vi "AutoWaitForArm_ORIG.vi"(8 "error in (no error)":errorcluster, 11 "TimeOut (s)":dbl=5.0) -> (0 "error out":errorcluster)   [LabVIEW 2020]
doc: "Wrapper class for auto do nothing and wait\nInput:\n -- error in -- Cluster \n -- time out -- Double -- how long to wait B4 quitting\nOutput:\n -- error out -- Cluster"
uses:
  <vilib>/Utility/semaphor.llb/Obtain Semaphore Reference.vi
  <vilib>/Rock Robotics/WPI/ThirdParty/JAS_Junk/TrajLib/Timer_Reset.vi
  <vilib>/Rock Robotics/WPI/ThirdParty/JAS_Junk/TrajLib/Trajectory_Library.lvlib
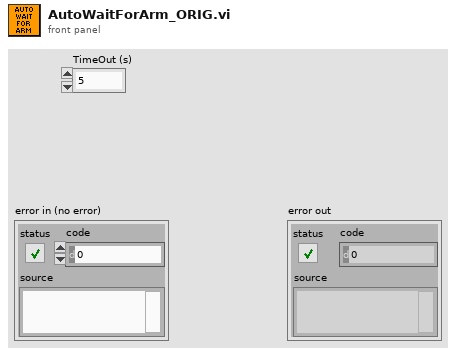
[diagram p1: front panel]
types:
  T1 = typedef "Trajectory_Library.lvlib/TIMER.ctl" = cluster{"StartTime":dbl, "Accumulated TIme":dbl, "Running":bool, "semaphore":T2}
  T2 = typedef "Semaphore RefNum" = refnum<k1>
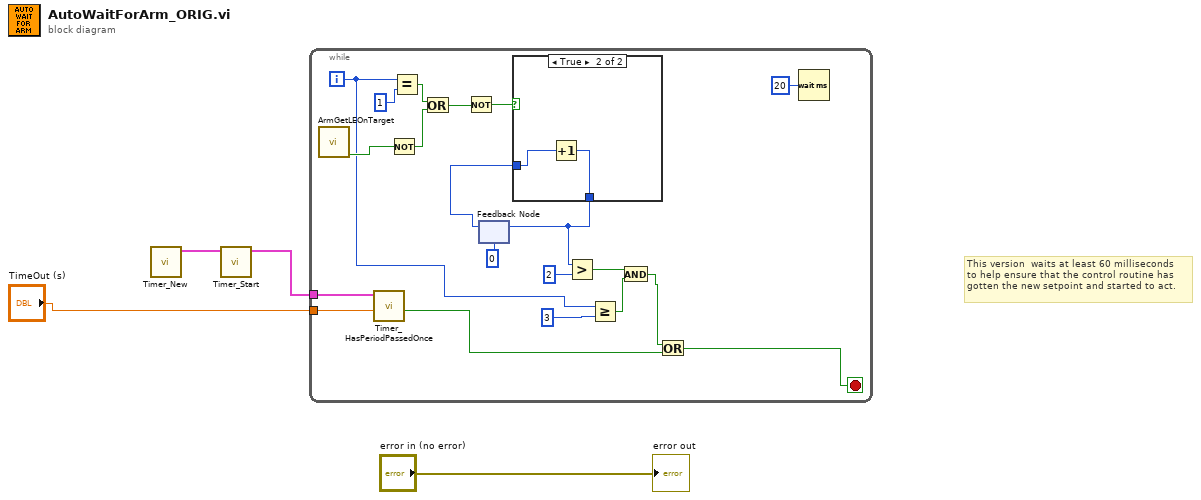
[diagram p0: block diagram]
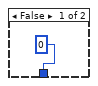
[diagram p2: hidden frame]
diagram:
  # "This version  waits at least 60 milliseconds\nto help ensure that the control routine has\ngotten the new setpoint and started to act."
  n1 = call <vilib>:"Timer_New.vi"() -> ("TIMER"=w3:T1)  [unwired: 11 in]
  n2 = call <vilib>:"Timer_Start.vi"("in Timer"=w3) -> ("out Timer"=w2:T1)  [unwired: 10 in]
  n3 = while {
    tunnel: w2 -> [w24]
    tunnel: "TimeOut (s)" -> [w23]
    i -> [w9]
    stop <- w20 stop-if-true
    n4 = call "ArmGetLEOnTarget.vi"() -> ("RLEOnTarget"=w14:bool)  [unwired: 11 in]
    n5 = call <vilib>:"Timer_HasPeriodPassedOnce.vi"("Period"=w23, "in Timer"=w24) -> ("Expired"=w21:bool)  [unwired: 7 in, 2 out]
    n6 = Not(x=w14) -> (.not. x?=w12:bool)
    n7 = Equal?(x=w9, y=1) -> (x = y?=w13:bool)
    n8 = Or(x=w13, y=w12) -> (x .or. y?=w11:bool)
    n9 = Not(x=w11) -> (.not. x?=w10:bool)
    n10 = feedback #1(0) -> (w15:i32)
    n11 = case shown="True" w10 {
      tunnel: [0 w26] -> w17
      tunnel: w15 -> [_ w27]
      frame False {
      }
      frame True {
        n12 = Increment(x=w27) -> (x+1=w26:i32)
      }
    }
    n13 = feedback-in #1(w17) -> ()
    n14 = Greater?(x=w17, y=2) -> (0:w7:bool)
    n15 = Greater Or Equal?(x=w9, y=3) -> (x >= y?=w6:bool)
    n16 = And(x=w7, y=w6) -> (x .and. y?=w5:bool)
    n17 = Or(x=w5, y=w21) -> (x .or. y?=w20:bool)
    n18 = Wait (ms)(milliseconds to wait=u32 20) -> ()  [unwired: 1 out]
  }
  "error out" <- "error in (no error)"
